vi "Variant_ExtractClusterElements.vi"(11 "Cluster":variant) -> (2 "name":string, 3 "Elements":variant[](array[variant]))   [LabVIEW 2013]
uses:
  TypeDescriptor/TypeDescriptor_GetPString.vi
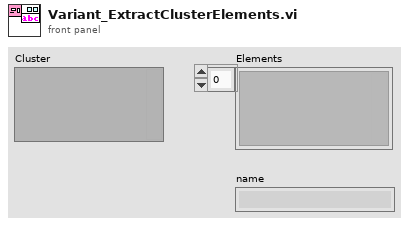
[diagram p1: front panel]
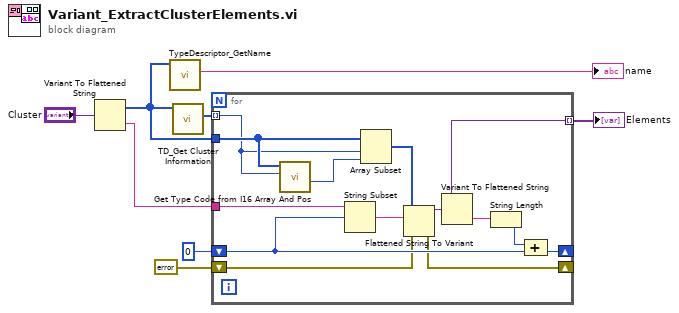
[diagram p0: block diagram]
diagram:
  n1 = Variant To Flattened String(Variant="Cluster") -> (data string=w8:string, 1:w2:i16[])
  n2 = call "TypeDescriptor_GetName.vi"("type descriptor"=w2) -> ("name"=→"name":string)  [unwired: 8 in, 2 out]
  n3 = call <vilib>:"TD_Get Cluster Information.vi"("Type descriptor"=w2) -> ("Contained TD Offsets"=w6:i32[])  [unwired: 9 in, 1 out]
  n4 = for {
    tunnel: w2 -> [w12]
    shift-right: [w16] -> _
    shift-left: 0 -> [w17]
    tunnel: w8 -> [w21]
    tunnel: [w15] -> w3 mode=indexing
    shift-right: [w13] -> _
    shift-left: errorcluster {"status"=FALSE, "code"=0, "source"=""} ("error out") -> [w14]
    tunnel: w6 -> [w10] mode=indexing
    n5 = call <vilib>:"Get Type Code from I16 Array And Pos.vi"("Pos in Type Descriptor (0)"=w10, "Type descriptor"=w12) -> ("Size (Words)"=w11:i32)  [unwired: 7 in, 2 out]
    n6 = String Subset(string=w21, offset (0)=w17) -> (substring=w20:string)  [unwired: 1 in]
    n7 = Array Subset(array=w12, index=w10, length=w11) -> (w9:i16[])
    n8 = Flattened String To Variant(4:w14, 6:w20, 7:w9) -> (0:w13:errorcluster, 3:w15:variant)
    n9 = Variant To Flattened String(Variant=w15) -> (data string=w19:string)  [unwired: 1 out]
    n10 = String Length(string=w19) -> (length=w18:i32)
    n11 = Compound Arithmetic op=ADD(w18, w17) -> (w16:i32)
  }
  "Elements" <- w3
